vi "motors_set_position.vi"(8 "error in (no error)":errorcluster, 9 "Position (deg)":i32, 10 "Axis":T1, 11 "MotorController in":refnum<class "MotorController.lvclass">) -> (0 "error out":errorcluster, 3 "MotorController out":refnum<class "MotorController.lvclass">)   [LabVIEW 2019, in "MotorController.lvclass"]
uses:
  MotorController.lvclass
  Axes_enum_typedef.ctl
  MotorController.lvclass/MotorController.ctl
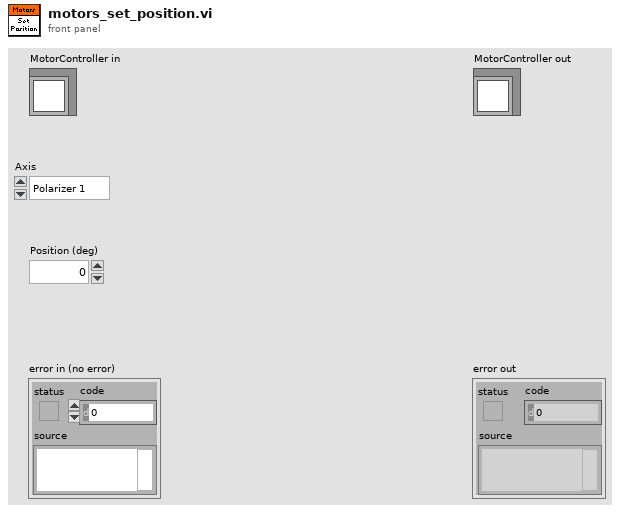
[diagram p1: front panel]
types:
  T1 = typedef "Axes_enum_typedef.ctl" = enum16{"Polarizer 1", "Polarizer 2", "Sample", "Stage"}
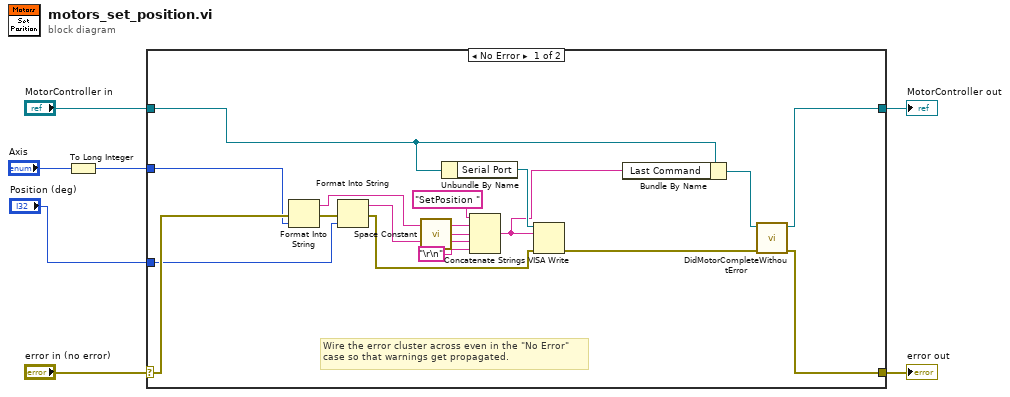
[diagram p0: block diagram]
diagram:
  n1 = To Long Integer(number="Axis") -> (32bit integer=w1:i32)
  n2 = case shown="No Error" "error in (no error)" {
    selector: "error in (no error)" -> [w14 w26]
    tunnel: [w13 w26] -> w6
    tunnel: [w15 w25] -> w4
    tunnel: "MotorController in" -> [w10 w25]
    tunnel: "Position (deg)" -> [w12 _]
    tunnel: w1 -> [w11 _]
    frame No Error {
      # "Wire the error cluster across even in the \"No Error\"\ncase so that warnings get propagated."
      n3 = Format Into String(error in=w14, w11) -> (resulting string=w22:string, error out=w24:errorcluster)  [unwired: 2 in]
      n4 = Format Into String(error in=w24, w12) -> (resulting string=w21:string, error out=w17:errorcluster)  [unwired: 2 in]
      n5 = call <vilib>:"Space Constant.vi"() -> ("String"=w20:string)
      n6 = Unbundle By Name(w10) -> ("Serial Port"=w18:refnum<visa-resource-name>)
      n7 = Concatenate Strings("SetPosition ", w22, w20, w21, "\r\n") -> (w8:string)
      n8 = VISA Write(VISA resource name=w18, write buffer=w8, error in (no error)=w17) -> (error out=w16:errorcluster)  [unwired: 2 out]
      n9 = Bundle By Name(cluster=w10, "Last Command"=w8) -> (w9:refnum<class "MotorController.lvclass">)
      n10 = call "DidMotorCompleteWithoutError.vi"("error in (no error)"=w16, "MotorController in"=w9) -> ("error out"=w13:errorcluster, "MotorController out"=w15:refnum<class "MotorController.lvclass">)  [unwired: 7 in, 1 out]
    }
    frame Error {
    }
  }
  "error out" <- w6
  "MotorController out" <- w4
